vi "Teleop.vi"(10 "Match Info":T1={"Autonomous Elapsed Seconds"=0.0, "TeleOp Elapsed Seconds"=0.0, "Disabled Elapsed Seconds"=0.0, "Visited Autonomous"=FALSE, "Visited TeleOp"=FALSE, "Visited Disabled"=FALSE, "Autonomous Settings"={"Autonomous Style"=enum."Independent", "VI Refnum"=refnum}}, 11 "Call Context":T2) -> ()   [LabVIEW 2015]
doc: "This VI is called for each TeleOp packet received from the DS where the robot is not disabled. It is often used to read from the joysticks and update I/O or to update setpoints for timed control loops. It should complete and return within 20 milliseconds or it may miss DS packets."
uses:
  <vilib>/Rock Robotics/WPI/DriverStation/WPI_DriverStationDerivedRobotMode.ctl
  <vilib>/Rock Robotics/WPI/DriverStation/WPI_DriverStationMatch Info.ctl
  <vilib>/Rock Robotics/WPI/Solenoid/WPI_SolenoidValue.ctl
  <vilib>/Rock Robotics/WPI/Utilities/WPI_GetSetVariantRefNum.vi
  <vilib>/Rock Robotics/WPI/Solenoid/WPI_SolenoidSetEnum.vi
  <vilib>/Rock Robotics/Network Tables/SD Write Boolean Array.vi
  <vilib>/Rock Robotics/Network Tables/SD Write Numeric Array.vi
  <vilib>/Rock Robotics/Network Tables/SD Read Boolean.vi
  <vilib>/Rock Robotics/Network Tables/SD Read Number.vi
panel:
  out "Sample Slider 0":dbl(slide) scale=0.0..5.0
  out "Sample Boolean 1":bool
  out "Sample Boolean 0":bool
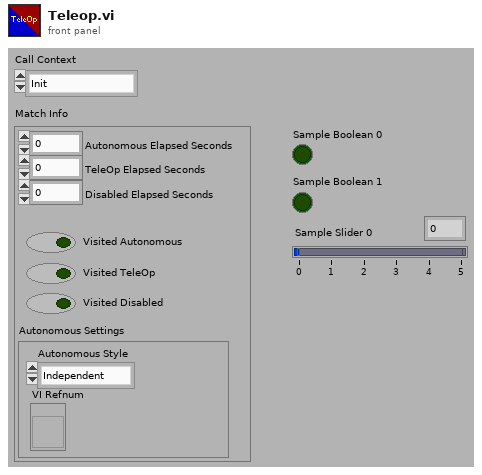
[diagram p1: front panel]
types:
  T1 = typedef "WPI_DriverStationMatch Info.ctl" = cluster{"Autonomous Elapsed Seconds":dbl, "TeleOp Elapsed Seconds":dbl, "Disabled Elapsed Seconds":dbl, "Visited Autonomous":bool, "Visited TeleOp":bool, "Visited Disabled":bool, "Autonomous Settings":cluster{"Autonomous Style":enum16{"Iterative", "Independent"}, "VI Refnum":refnum<vi>}}
  T2 = typedef "WPI_DriverStationDerivedRobotMode.ctl" = enum16{"Init", "Execute", "Stop"}
  T3 = typedef "WPI_JoystickDevRef.ctl" = cluster{"Device":T4}
  T4 = typedef "WPI_JoystickDeviceEnum.ctl" = enum16{"USB 0", "USB 1", "USB 2", "USB 3", "USB 4", "USB 5"}
  T5 = typedef "WPI_RobotDriveDevRef.ctl" = cluster{"DevStatus":errorcluster, "Motors[]":T6[], "Square Inputs":bool, "Max Output":dbl}
  T6 = typedef "WPI_MotorControlDeviceRef.ctl" = cluster{"DeviceStatus":errorcluster, "Type":T7, "PWM":cluster{"PWM Channel":T8, "DeadBand":T9}, "CAN":cluster{"Device Number":u8, "Control Mode":T10, "Semaphore":T11, "Max Vout":dbl, "TalonSRX Control Mode":T12}, "Invert":bool}
  T7 = typedef "WPI_MotorControlType.ctl" = enum16{"PWM", "CAN", "CANTalonSRX"}
  T8 = typedef "FPGA_DIOPWMChannel.ctl" = enum8{"PWM 0", "PWM 1", "PWM 2", "PWM 3", "PWM 4", "PWM 5", "PWM 6", "PWM 7", "PWM 8", "PWM 9", "PWM MXP 0", "PWM MXP 1", "PWM MXP 2", "PWM MXP 3", "PWM MXP 4", "PWM MXP 5", "PWM MXP 6", "PWM MXP 7", "PWM MXP 8", "PWM MXP 9", "Invalid"}
  T9 = typedef "WPI_PWMDeadband.ctl" = cluster{"Name":string, "maxPositivePwm":i32, "minPositivePwm":i32, "centerPwm":i32, "maxNegativePwm":i32, "minNegativePwm":i32, "angularRange":u16}
  T10 = typedef "WPI_CANJaguar_ControlMode.ctl" = enum8{"Percent VBus", "Current", "Speed", "Position", "Voltage"}
  T11 = typedef "Semaphore RefNum" = refnum<k1>
  T12 = typedef "WPI_CANTalonSRX_APIControlMode.ctl" = enum8{"Percent VBus", "Speed", "Position", "Slave", "Unchanged / Invalid", "Voltage Compensation", "Current", "Motion Profile"}
  T13 = cluster{"Buttons[0]":bool, "Buttons[1]":bool, "Buttons[2]":bool, "Buttons[3]":bool, "Buttons[4]":bool, "Buttons[5]":bool, "Buttons[6]":bool, "Buttons[7]":bool, "Buttons[8]":bool}
  T14 = typedef "WPI_SolenoidValue.ctl" = enum16{"Off", "On", "Forward", "Reverse"}
  T15 = typedef "WPI_SolenoidDevRef.ctl" = cluster{"DevStatus":errorcluster, "Pneumatics Control Module":u8, "Forward Solenoid Channel":T16, "Reverse Solenoid Channel":T16}
  T16 = typedef "WPI_SolenoidChannel.ctl" = enum8{"Solenoid 0", "Solenoid 1", "Solenoid 2", "Solenoid 3", "Solenoid 4", "Solenoid 5", "Solenoid 6", "Solenoid 7", "Invalid"}
  T17 = typedef "WPI_AOChannelDevRef.ctl" = cluster{"DevStatus":errorcluster, "AO Channel":T18}
  T18 = typedef "WPI_AnalogOutputChannel.ctl" = enum8{"AO MXP 0", "AO MXP 1", "Invalid"}
  T19 = typedef "WPI_ServoDeviceRef.ctl" = cluster{"DeviceStatus":errorcluster, "PWM Channel":T8, "DeadBand":T9}
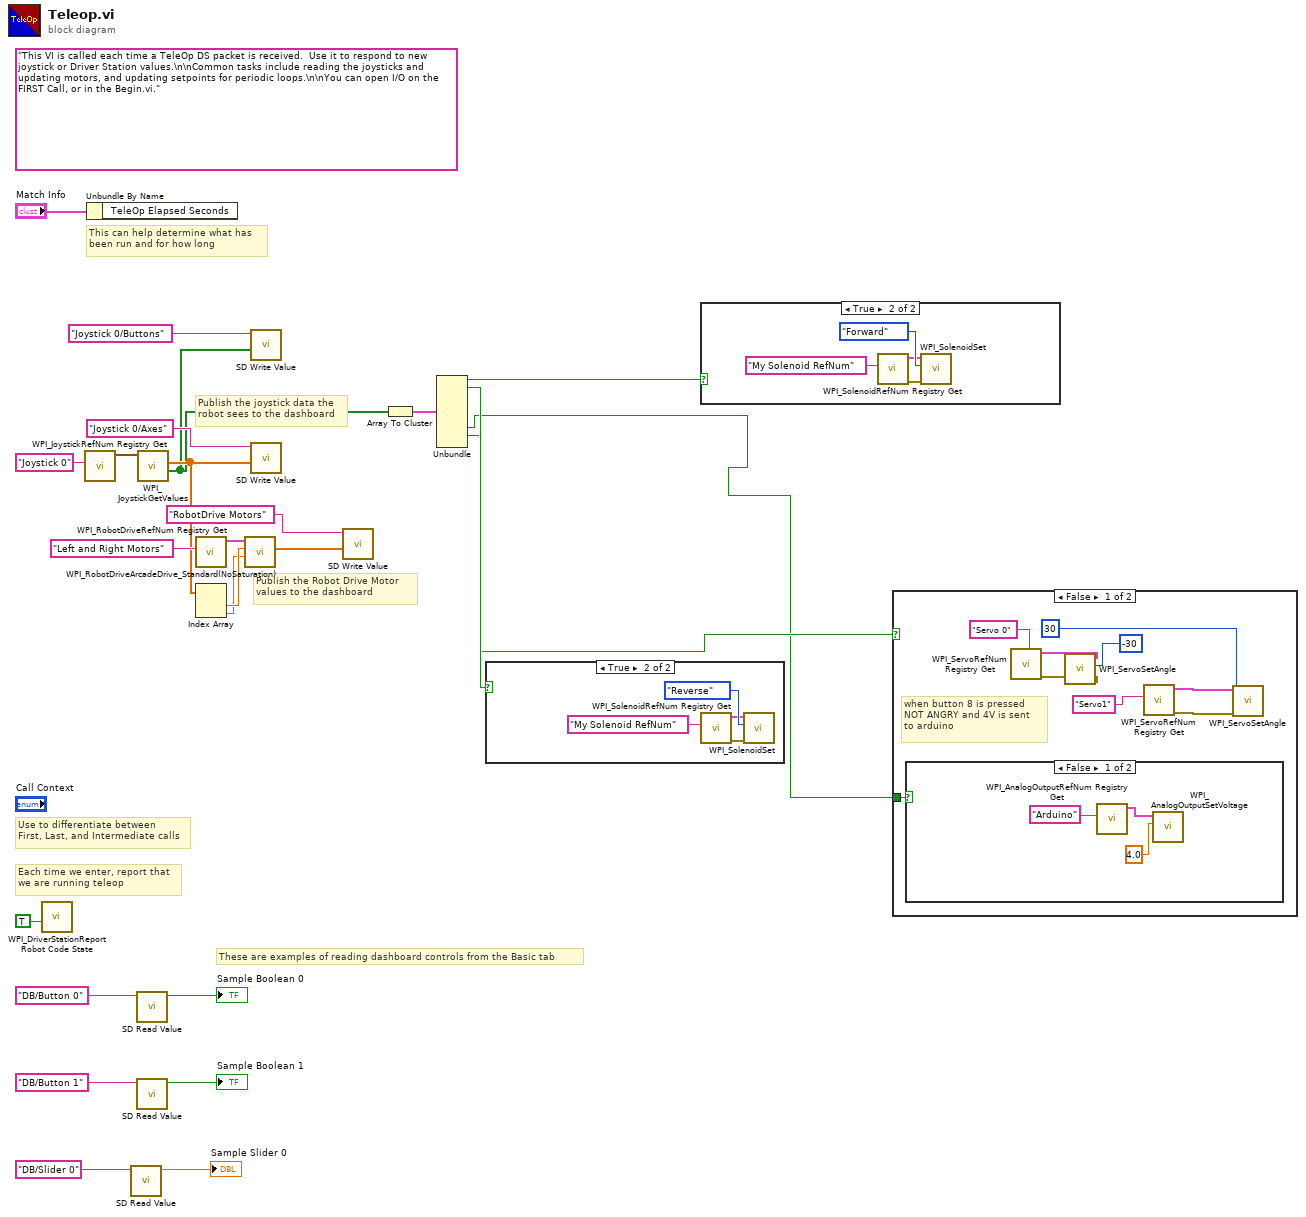
[diagram p0: block diagram]
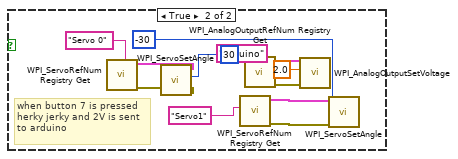
[diagram p2: hidden frame]
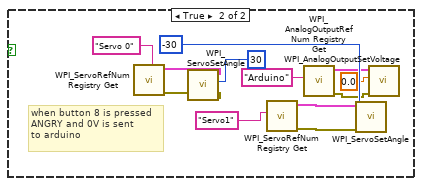
[diagram p3: hidden frame]
diagram:
  (unwired) "This VI is called each time a TeleOp DS packet is received.  Use it to respond to new joystick or Driver Station values.\n\nCommon tasks include reading the joysticks and updating motors, and updating setpoints for periodic loops.\n\nYou can open I/O on the FIRST Call, or in the Begin.vi."
  # "These are examples of reading dashboard controls from the Basic tab"
  # "Publish the Robot Drive Motor\nvalues to the dashboard"
  # "Publish the joystick data the\nrobot sees to the dashboard"
  # "Each time we enter, report that\nwe are running teleop"
  # "Use to differentiate between\nFirst, Last, and Intermediate calls"
  # "This can help determine what has\nbeen run and for how long"
  n1 = call <vilib>:"WPI_DriverStationReport Robot Code State.vi"("TeleOp"=TRUE ("Autonomous")) -> ()  [unwired: 10 in, 1 out]
  n2 = call <vilib>:"WPI_JoystickRefNum Registry Get.vi"("refnum name"="Joystick 0") -> ("JoystickDevRef"=w21:T3)  [unwired: 1 in, 9 out]
  n3 = Unbundle By Name("Match Info") -> ()  [unwired: 1 out]
  n4 = call-poly <vilib>:"SD Read Value.vi"("Name"="DB/Slider 0" ("refnum name")) -> ("Numeric"=→"Sample Slider 0":dbl)  [unwired: 8 in, 2 out]
  n5 = call-poly <vilib>:"SD Read Value.vi"("Name"="DB/Button 0" ("refnum name")) -> ("Boolean"=→"Sample Boolean 0":bool)  [unwired: 8 in, 2 out]
  n6 = call-poly <vilib>:"SD Read Value.vi"("Name"="DB/Button 1" ("refnum name")) -> ("Boolean"=→"Sample Boolean 1":bool)  [unwired: 8 in, 2 out]
  n7 = call <vilib>:"WPI_JoystickGetValues.vi"("JoystickDevRef"=w21) -> ("Buttons"=w8:bool[], "Axes"=w10:dbl[])  [unwired: 6 in, 3 out]
  n8 = call <vilib>:"WPI_RobotDriveRefNum Registry Get.vi"("refnum name"="Left and Right Motors") -> ("RobotDriveDevRef"=w23:T5)  [unwired: 1 in, 9 out]
  n9 = Index Array(array=w10) -> (element #1=w4:dbl, element #2=w3:dbl)  [unwired: 2 in]
  n10 = call <vilib>:"WPI_RobotDriveArcadeDrive_Standard(NoSaturation).vi"("Y axis value"=w3, "X axis value"=w4, "RobotDriveDevRef"=w23) -> ("Motor Values"=w12:dbl[])  [unwired: 1 in, 7 out]
  n11 = call-poly <vilib>:"SD Write Value.vi"("Boolean Array"=w8, "Name"="Joystick 0/Buttons") -> ()  [unwired: 8 in, 2 out]
  n12 = call-poly <vilib>:"SD Write Value.vi"("Numeric Array"=w10, "Name"="Joystick 0/Axes") -> ()  [unwired: 8 in, 2 out]
  n13 = call-poly <vilib>:"SD Write Value.vi"("Numeric Array"=w12, "Name"="RobotDrive Motors") -> ()  [unwired: 8 in, 2 out]
  n14 = Array To Cluster(array=w8) -> (cluster=w7:T13)
  n15 = Unbundle(w7) -> ("Buttons[0]"=w6:bool, "Buttons[1]"=w5:bool, "Buttons[6]"=w1:bool, "Buttons[7]"=w2:bool)  [unwired: 5 out]
  n16 = case shown="True" w5 {
    frame False {
    }
    frame True {
      n17 = call <vilib>:"WPI_SolenoidRefNum Registry Get.vi"("refnum name"="My Solenoid RefNum") -> ("error out"=w27:errorcluster, "SolenoidDevRef"=w28:T15)  [unwired: 9 in]
      n18 = call-poly <vilib>:"WPI_SolenoidSet.vi"("error in (no error)"=w27, "Value"=WPI_SolenoidValue."Reverse", "SolenoidDevRef"=w28) -> ()  [unwired: 7 in, 2 out]
    }
  }
  n19 = case shown="True" w6 {
    frame False {
    }
    frame True {
      n20 = call <vilib>:"WPI_SolenoidRefNum Registry Get.vi"("refnum name"="My Solenoid RefNum") -> ("error out"=w31:errorcluster, "SolenoidDevRef"=w32:T15)  [unwired: 9 in]
      n21 = call-poly <vilib>:"WPI_SolenoidSet.vi"("error in (no error)"=w31, "Value"=WPI_SolenoidValue."Forward", "SolenoidDevRef"=w32) -> ()  [unwired: 7 in, 2 out]
    }
  }
  n22 = case shown="False" w2 {
    tunnel: w1 -> [w34 _]
    frame False {
      # "when button 8 is pressed\nNOT ANGRY and 4V is sent\nto arduino"
      n23 = case shown="False" w34 {
        frame False {
          n24 = call <vilib>:"WPI_AnalogOutputRefNum Registry Get.vi"("refnum name"="Arduino") -> ("AODeviceRef"=w45:T17)  [unwired: 9 in, 1 out]
          n25 = call <vilib>:"WPI_AnalogOutputSetVoltage.vi"("Voltage"=4.0, "AODeviceRef"=w45) -> ()  [unwired: 8 in, 2 out]
        }
        frame True {
          # "when button 7 is pressed\nherky jerky and 2V is sent\nto arduino"
          n26 = call <vilib>:"WPI_ServoRefNum Registry Get.vi"("refnum name"="Servo 0") -> ("error out"=w56:errorcluster, "ServoDeviceRef"=w57:T19)  [unwired: 9 in]
          n27 = call <vilib>:"WPI_ServoSetAngle.vi"("error in (no error)"=w56, "Angle"=30, "ServoDeviceRef"=w57) -> ()  [unwired: 7 in, 2 out]
          n28 = call <vilib>:"WPI_ServoRefNum Registry Get.vi"("refnum name"="Servo1") -> ("error out"=w52:errorcluster, "ServoDeviceRef"=w53:T19)  [unwired: 9 in]
          n29 = call <vilib>:"WPI_AnalogOutputRefNum Registry Get.vi"("refnum name"="Arduino") -> ("error out"=w49:errorcluster, "AODeviceRef"=w48:T17)  [unwired: 9 in]
          n30 = call <vilib>:"WPI_AnalogOutputSetVoltage.vi"("error in (no error)"=w49, "Voltage"=2.0, "AODeviceRef"=w48) -> ()  [unwired: 7 in, 2 out]
          n31 = call <vilib>:"WPI_ServoSetAngle.vi"("error in (no error)"=w52, "Angle"=-30, "ServoDeviceRef"=w53) -> ()  [unwired: 7 in, 2 out]
        }
      }
      n32 = call <vilib>:"WPI_ServoRefNum Registry Get.vi"("refnum name"="Servo 0") -> ("error out"=w41:errorcluster, "ServoDeviceRef"=w42:T19)  [unwired: 9 in]
      n33 = call <vilib>:"WPI_ServoSetAngle.vi"("error in (no error)"=w41, "Angle"=-30, "ServoDeviceRef"=w42) -> ()  [unwired: 7 in, 2 out]
      n34 = call <vilib>:"WPI_ServoRefNum Registry Get.vi"("refnum name"="Servo1") -> ("error out"=w37:errorcluster, "ServoDeviceRef"=w38:T19)  [unwired: 9 in]
      n35 = call <vilib>:"WPI_ServoSetAngle.vi"("error in (no error)"=w37, "Angle"=30, "ServoDeviceRef"=w38) -> ()  [unwired: 7 in, 2 out]
    }
    frame True {
      # "when button 8 is pressed\nANGRY and 0V is sent\nto arduino"
      n36 = call <vilib>:"WPI_ServoRefNum Registry Get.vi"("refnum name"="Servo 0") -> ("error out"=w68:errorcluster, "ServoDeviceRef"=w69:T19)  [unwired: 9 in]
      n37 = call <vilib>:"WPI_ServoSetAngle.vi"("error in (no error)"=w68, "Angle"=30, "ServoDeviceRef"=w69) -> ()  [unwired: 7 in, 2 out]
      n38 = call <vilib>:"WPI_ServoRefNum Registry Get.vi"("refnum name"="Servo1") -> ("error out"=w64:errorcluster, "ServoDeviceRef"=w65:T19)  [unwired: 9 in]
      n39 = call <vilib>:"WPI_AnalogOutputRefNum Registry Get.vi"("refnum name"="Arduino") -> ("error out"=w58:errorcluster, "AODeviceRef"=w60:T17)  [unwired: 9 in]
      n40 = call <vilib>:"WPI_ServoSetAngle.vi"("error in (no error)"=w64, "Angle"=-30, "ServoDeviceRef"=w65) -> ()  [unwired: 7 in, 2 out]
      n41 = call <vilib>:"WPI_AnalogOutputSetVoltage.vi"("error in (no error)"=w58, "Voltage"=0.0, "AODeviceRef"=w60) -> ()  [unwired: 7 in, 2 out]
    }
  }
